vi "get shared data ref.vi"(8 "error in (no error)":errorcluster, 11 "Item Ref in":T2 format="%.0x") -> (0 "error out":errorcluster, 2 "shared data ref":T1, 3 "Item Ref out":T2 format="%.0x")   [LabVIEW 2017, in "DSF System Explorer.lvlib"]
uses:
  DSF System Explorer.lvlib
  <vilib>/NI Veristand/Custom Device API/Custom Device Item Ref.ctl
  shared data ref.ctl
  shared data.ctl
  DSF Core.lvlibp/Classes/Configuration/Configuration Session.lvclass
  Shared/DSF Shared.lvlib
  <vilib>/NI Veristand/Custom Device API/Custom Device API.lvlib
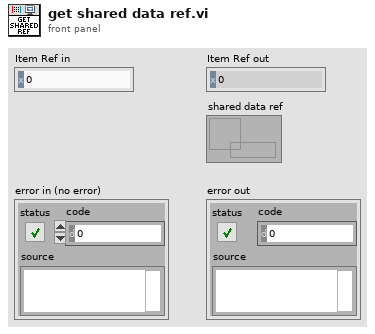
[diagram p1: front panel]
types:
  T1 = typedef "DSF System Explorer.lvlib/shared data ref.ctl" = refnum<data-value>
  T2 = typedef "Custom Device API.lvlib/Custom Device Item Ref.ctl" = u64
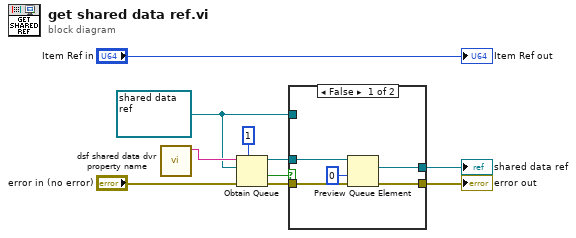
[diagram p0: block diagram]
diagram:
  w2 = T1 refnum ("shared data ref 2")
  n1 = call "dsf shared data dvr property name.vi"() -> ("shared data dvr property name"=w7:string)  [unwired: 11 in]
  n2 = Obtain Queue(max queue size (-1, unlimited)=1, name (unnamed)=w7, element data type=w2, error in (no error)="error in (no error)") -> (queue out=w8:refnum<queue>, created new?=w5:bool, error out=w9:errorcluster)  [unwired: 1 in]
  n3 = case shown="False" w5 {
    tunnel: w9 -> [w14 w17]
    tunnel: w8 -> [w15 _]
    tunnel: w2 -> [_ w16]
    tunnel: [w12 w17] -> w3
    tunnel: [w13 w16] -> w1
    frame False {
      n4 = Preview Queue Element(queue=w15, timeout in ms (-1)=0, error in (no error)=w14) -> (element=w13:T1, error out=w12:errorcluster)  [unwired: 2 out]
    }
    frame True {
    }
  }
  "error out" <- w3
  "shared data ref" <- w1
  "Item Ref out" <- "Item Ref in"
